vi "盐度补偿值读取.vi"(8 "Error in":errorcluster caption="Error in (no error)", 11 "MB session in":refnum<class "MB_Master.lvclass">) -> (0 "error out":errorcluster, 2 "盐度补偿值":sgl, 3 "MB session out":refnum<class "MB_Master.lvclass">)   [LabVIEW 2016, in "斯坦道氨氮.lvlib"]
uses:
  <vilib>/Plasmionique/MB Master/MB_Master/MB_Master.lvclass
  <vilib>/Plasmionique/MB Master/MB Master.lvlib
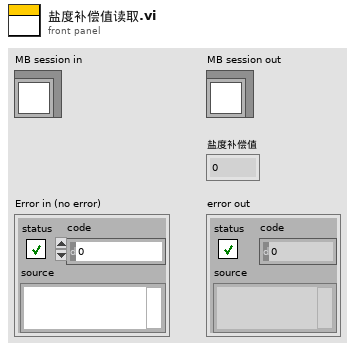
[diagram p1: front panel]
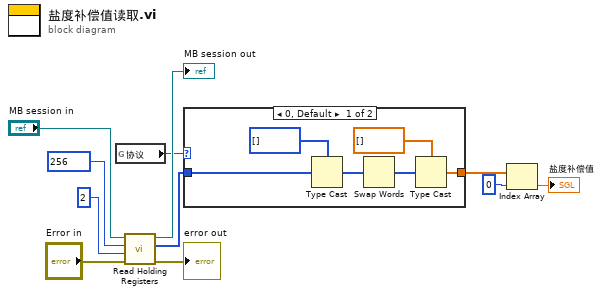
[diagram p0: block diagram]
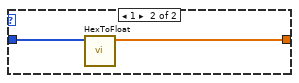
[diagram p2: hidden frame]
diagram:
  n1 = global read "总磷总氮断电保存全局变量.vi" "协议"() -> (w1:u16)
  n2 = call <vilib>:"Read Holding Registers.vi"("error in (no error)"="Error in", "quantity"=u16 2, "starting address"=u16 256, "MB session in"="MB session in") -> ("error out"=→"error out":errorcluster, "Registers"=w5:u16[], "MB session out"=→"MB session out":refnum<class "MB_Master.lvclass">)  [unwired: 5 in]
  n3 = case shown="0, Default" w1 {
    tunnel: w5 -> [w13 w19]
    tunnel: [w12 w18] -> w4
    frame 0, Default {
      n4 = Type Cast(type=u32[] [], x=w13) -> (*(type *) &x=w15:u32[])
      n5 = Swap Words(1:w15) -> (0:w14:u32[])
      n6 = Type Cast(type=sgl[] [], x=w14) -> (*(type *) &x=w12:sgl[])
    }
    frame 1 {
      n7 = call "HexToFloat.vi"("数组"=w19) -> ("FLOAT"=w18:sgl[])  [unwired: 10 in]
    }
  }
  n8 = Index Array(array=w4, index=0 ("索引")) -> (element=→"盐度补偿值":sgl)
